vi "SigInfo _FGV.vi"(7 "Function (Read)":enum16{"Read", "Write"}(ring), 8 "error in (no error)":errorcluster, 11 "mzInfo in":refnum<class "SigInfo.lvclass">) -> (0 "error out":errorcluster, 3 "mzInfo out":refnum<class "SigInfo.lvclass">)   [LabVIEW 2018, in "SigInfo.lvclass"]
uses:
  SigInfo.lvclass
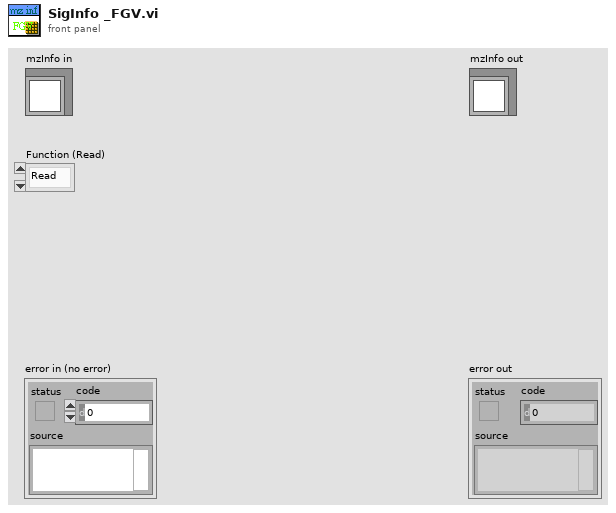
[diagram p1: front panel]
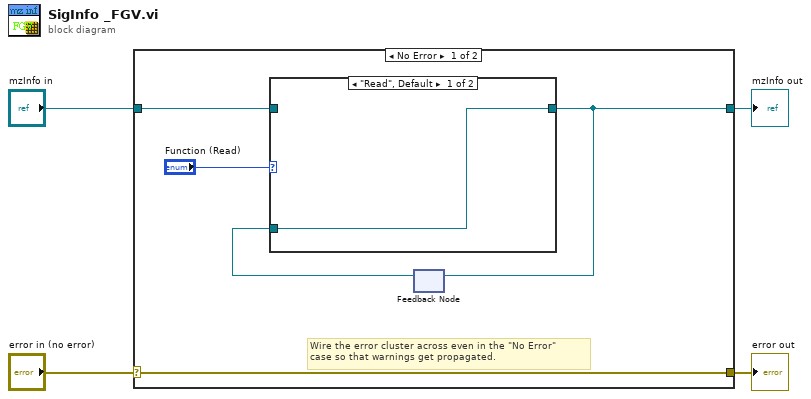
[diagram p0: block diagram]
diagram:
  n1 = case shown="No Error" "error in (no error)" {
    selector: "error in (no error)" -> [w9 w13]
    tunnel: [w9 w13] -> w3
    tunnel: [w6 w12] -> w1
    tunnel: "mzInfo in" -> [w8 w12]
    frame No Error {
      # "Wire the error cluster across even in the \"No Error\"\ncase so that warnings get propagated."
      n2 = feedback #1() -> (w5:refnum<class "SigInfo.lvclass">)  [unwired: 1 in]
      n3 = case shown="\"Read\", Default" "Function (Read)" {
        tunnel: w8 -> [_ w11]
        tunnel: [w10 w11] -> w6
        tunnel: w5 -> [w10 _]
        frame "Read", Default {
        }
        frame "Write" {
        }
      }
      n4 = feedback-in #1(w6) -> ()
    }
    frame Error {
    }
  }
  "error out" <- w3
  "mzInfo out" <- w1
